vi "Build Channel Cluster Array.vi"() -> (3 "Channels out":cluster{"Channels":T1[]})   [LabVIEW 2023, in "Cycler Cluster - 6 Channel.lvclass"]
uses:
  Cycler Cluster - 6 Channel.lvclass
  Utilities/Channel.ctl
  Cycler Cluster - 6 Channel.lvclass/Cycler Cluster - 6 Channel.ctl
  Utilities/Utilities.lvlib
panel:
  in  "Cycler Cluster - 24 Channel.lvclass":refnum<class "Cycler Cluster - 6 Channel.lvclass">
  in  "Channels in":cluster{"Channels":T1[]}
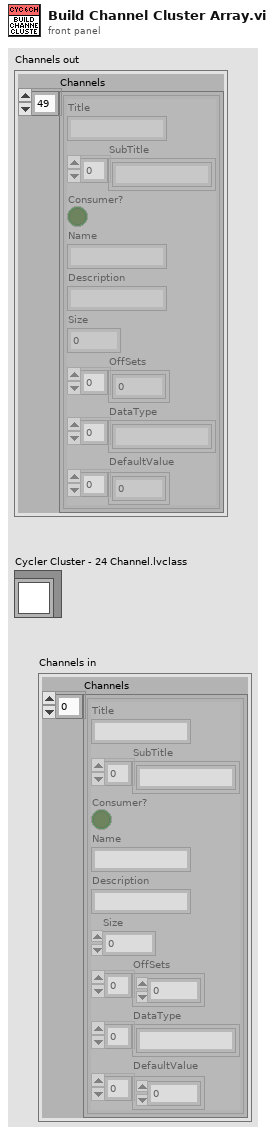
[diagram p1: front panel]
types:
  T1 = typedef "Utilities.lvlib/Channel.ctl" = cluster{"Title":string, "SubTitle":string[], "Consumer?":bool, "Name":string, "Description":string, "Size":i32, "OffSets":i32[], "DataType":string[], "DefaultValue":dbl[]}
  T2 = cluster{"Error.ch01.STS":i32, "OutputEnable.ch01.STS":i32, "ControlMode.ch01.STS":u16, "Voltage.ch01.AV":dbl, "Current.ch01.AV":dbl, "Power.ch01.AV":dbl, "VoltageNominal.ch01.AV":dbl, "CurrentNominal.ch01.AV":dbl, "PowerNominal.ch01.AV":dbl, "ParameterSet.ch01.STS":i32}
  T3 = cluster{"ErrorAcknowledge.ch02.ACT":bool, "OutputEnable.ch02.ACT":bool, "ControlMode.ch02.CTL":u16, "Voltage.ch02.SP":dbl, "VoltageMIN.ch02.SP":dbl, "VoltageMAX.ch02.SP":dbl, "VoltageGrad.ch02.SP":dbl, "Current.ch02.SP":dbl, "CurrentMIN.ch02.SP":dbl, "CurrentMAX.ch02.SP":dbl, "CurrentGrad.ch02.SP":dbl, "Power.ch02.SP":dbl, "PowerMIN.ch02.SP":dbl, "PowerMAX.ch02.SP":dbl, "PowerGrad.ch02.SP":dbl, "ParameterSet.ch02.CTL":i32}
  T4 = cluster{"Error.ch02.STS":i32, "OutputEnable.ch02.STS":i32, "ControlMode.ch02.STS":u16, "Voltage.ch02.AV":dbl, "Current.ch02.AV":dbl, "Power.ch02.AV":dbl, "VoltageNominal.ch02.AV":dbl, "CurrentNominal.ch02.AV":dbl, "PowerNominal.ch02.AV":dbl, "ParameterSet.ch02.STS":i32}
  T5 = cluster{"ErrorAcknowledge.ch03.ACT":bool, "OutputEnable.ch03.ACT":bool, "ControlMode.ch03.CTL":u16, "Voltage.ch03.SP":dbl, "VoltageMIN.ch03.SP":dbl, "VoltageMAX.ch03.SP":dbl, "VoltageGrad.ch03.SP":dbl, "Current.ch03.SP":dbl, "CurrentMIN.ch03.SP":dbl, "CurrentMAX.ch03.SP":dbl, "CurrentGrad.ch03.SP":dbl, "Power.ch03.SP":dbl, "PowerMIN.ch03.SP":dbl, "PowerMAX.ch03.SP":dbl, "PowerGrad.ch03.SP":dbl, "ParameterSet.ch03.CTL":i32}
  T6 = cluster{"Error.ch03.STS":i32, "OutputEnable.ch03.STS":i32, "ControlMode.ch03.STS":u16, "Voltage.ch03.AV":dbl, "Current.ch03.AV":dbl, "Power.ch03.AV":dbl, "VoltageNominal.ch03.AV":dbl, "CurrentNominal.ch03.AV":dbl, "PowerNominal.ch03.AV":dbl, "ParameterSet.ch03.STS":i32}
  T7 = cluster{"ErrorAcknowledge.ch04.ACT":bool, "OutputEnable.ch04.ACT":bool, "ControlMode.ch04.CTL":u16, "Voltage.ch04.SP":dbl, "VoltageMIN.ch04.SP":dbl, "VoltageMAX.ch04.SP":dbl, "VoltageGrad.ch04.SP":dbl, "Current.ch04.SP":dbl, "CurrentMIN.ch04.SP":dbl, "CurrentMAX.ch04.SP":dbl, "CurrentGrad.ch04.SP":dbl, "Power.ch04.SP":dbl, "PowerMIN.ch04.SP":dbl, "PowerMAX.ch04.SP":dbl, "PowerGrad.ch04.SP":dbl, "ParameterSet.ch04.CTL":i32}
  T8 = cluster{"Error.ch04.STS":i32, "OutputEnable.ch04.STS":i32, "ControlMode.ch04.STS":u16, "Voltage.ch04.AV":dbl, "Current.ch04.AV":dbl, "Power.ch04.AV":dbl, "VoltageNominal.ch04.AV":dbl, "CurrentNominal.ch04.AV":dbl, "PowerNominal.ch04.AV":dbl, "ParameterSet.ch04.STS":i32}
  T9 = cluster{"ErrorAcknowledge.ch05.ACT":bool, "OutputEnable.ch05.ACT":bool, "ControlMode.ch05.CTL":u16, "Voltage.ch05.SP":dbl, "VoltageMIN.ch05.SP":dbl, "VoltageMAX.ch05.SP":dbl, "VoltageGrad.ch05.SP":dbl, "Current.ch05.SP":dbl, "CurrentMIN.ch05.SP":dbl, "CurrentMAX.ch05.SP":dbl, "CurrentGrad.ch05.SP":dbl, "Power.ch05.SP":dbl, "PowerMIN.ch05.SP":dbl, "PowerMAX.ch05.SP":dbl, "PowerGrad.ch05.SP":dbl, "ParameterSet.ch05.CTL":i32}
  T10 = cluster{"Error.ch05.STS":i32, "OutputEnable.ch05.STS":i32, "ControlMode.ch05.STS":u16, "Voltage.ch05.AV":dbl, "Current.ch05.AV":dbl, "Power.ch05.AV":dbl, "VoltageNominal.ch05.AV":dbl, "CurrentNominal.ch05.AV":dbl, "PowerNominal.ch05.AV":dbl, "ParameterSet.ch05.STS":i32}
  T11 = cluster{"ErrorAcknowledge.ch06.ACT":bool, "OutputEnable.ch06.ACT":bool, "ControlMode.ch06.CTL":u16, "Voltage.ch06.SP":dbl, "VoltageMIN.ch06.SP":dbl, "VoltageMAX.ch06.SP":dbl, "VoltageGrad.ch06.SP":dbl, "Current.ch06.SP":dbl, "CurrentMIN.ch06.SP":dbl, "CurrentMAX.ch06.SP":dbl, "CurrentGrad.ch06.SP":dbl, "Power.ch06.SP":dbl, "PowerMIN.ch06.SP":dbl, "PowerMAX.ch06.SP":dbl, "PowerGrad.ch06.SP":dbl, "ParameterSet.ch06.CTL":i32}
  T12 = cluster{"Error.ch06.STS":i32, "OutputEnable.ch06.STS":i32, "ControlMode.ch06.STS":u16, "Voltage.ch06.AV":dbl, "Current.ch06.AV":dbl, "Power.ch06.AV":dbl, "VoltageNominal.ch06.AV":dbl, "CurrentNominal.ch06.AV":dbl, "PowerNominal.ch06.AV":dbl, "ParameterSet.ch06.STS":i32}
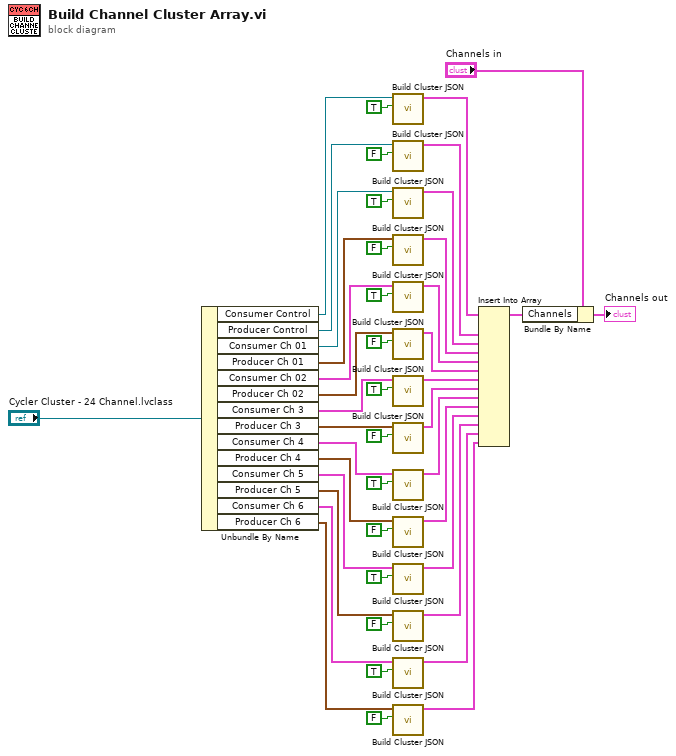
[diagram p0: block diagram]
diagram:
  n1 = Unbundle By Name("Cycler Cluster - 24 Channel.lvclass") -> ("Consumer Control"=w46:refnum<k21>, "Producer Control"=w45:refnum<k21>, "Consumer Ch 01"=w34:refnum<k21>, "Producer Ch 01"=w35:T2, "Consumer Ch 02"=w27:T3, "Producer Ch 02"=w26:T4, "Consumer Ch 3"=w16:T5, "Producer Ch 3"=w15:T6, "Consumer Ch 4"=w14:T7, "Producer Ch 4"=w13:T8, "Consumer Ch 5"=w12:T9, "Producer Ch 5"=w11:T10, "Consumer Ch 6"=w10:T11, "Producer Ch 6"=w9:T12)
  n2 = call "Build Cluster JSON.vi"("Consumer?"=TRUE, "Cluster"=w46) -> ("Array"=w42:T1[])  [unwired: 9 in]
  n3 = call "Build Cluster JSON.vi"("Consumer?"=FALSE, "Cluster"=w45) -> ("Array"=w41:T1[])  [unwired: 9 in]
  n4 = call "Build Cluster JSON.vi"("Consumer?"=TRUE, "Cluster"=w34) -> ("Array"=w33:T1[])  [unwired: 9 in]
  n5 = call "Build Cluster JSON.vi"("Consumer?"=FALSE, "Cluster"=w35) -> ("Array"=w32:T1[])  [unwired: 9 in]
  n6 = call "Build Cluster JSON.vi"("Consumer?"=TRUE, "Cluster"=w27) -> ("Array"=w29:T1[])  [unwired: 9 in]
  n7 = call "Build Cluster JSON.vi"("Consumer?"=FALSE, "Cluster"=w26) -> ("Array"=w28:T1[])  [unwired: 9 in]
  n8 = call "Build Cluster JSON.vi"("Consumer?"=TRUE, "Cluster"=w16) -> ("Array"=w8:T1[])  [unwired: 9 in]
  n9 = call "Build Cluster JSON.vi"("Consumer?"=FALSE, "Cluster"=w15) -> ("Array"=w7:T1[])  [unwired: 9 in]
  n10 = call "Build Cluster JSON.vi"("Consumer?"=TRUE, "Cluster"=w14) -> ("Array"=w6:T1[])  [unwired: 9 in]
  n11 = call "Build Cluster JSON.vi"("Consumer?"=FALSE, "Cluster"=w13) -> ("Array"=w5:T1[])  [unwired: 9 in]
  n12 = call "Build Cluster JSON.vi"("Consumer?"=TRUE, "Cluster"=w12) -> ("Array"=w4:T1[])  [unwired: 9 in]
  n13 = call "Build Cluster JSON.vi"("Consumer?"=FALSE, "Cluster"=w11) -> ("Array"=w3:T1[])  [unwired: 9 in]
  n14 = call "Build Cluster JSON.vi"("Consumer?"=TRUE, "Cluster"=w10) -> ("Array"=w2:T1[])  [unwired: 9 in]
  n15 = call "Build Cluster JSON.vi"("Consumer?"=FALSE, "Cluster"=w9) -> ("Array"=w1:T1[])  [unwired: 9 in]
  n16 = Insert Into Array(array=w42, new element #1=w41, new element #2=w33, new element #3=w32, new element #4=w29, new element #5=w28, new element #6=w8, new element #7=w7, new element #8=w6, new element #9=w5, new element #10=w4, new element #11=w3, new element #12=w2, new element #13=w1) -> (w39:T1[])  [unwired: 1 in]
  n17 = Bundle By Name(cluster="Channels in", "Channels"=w39) -> (→"Channels out":cluster{"Channels":T1[]})
